vi "XOR Plain Text with Random String.vi"() -> ()   [LabVIEW 2016]
panel:
  out "Plaintext Distribution":dynamicdata(graph)=[{"t0"=timestamp(0.5 s since 1904-01-01), "dt"=1.0, "Y"=[0.0, 0.0, 0.0, 0.0, 0.0, 0.0, 0.0, 0.0, 0.0, 0.0, 0.0, 0.0, 0.0, 0.0, 0.0, 0.0, 0.0, 0.0, 0.0, 0.0, 0.0, 0.0, 0.0, 0.0, 0.0, 0.0, 0.0, 0.0, 0.0, 0.0, 0.0, 0.0, 68.0, 0.0, 0.0, 0.0, 0.0, 0.0, 0.0, 0.0, 0.0, 0.0, 0.0, 0.0, 4.0, 0.0, 4.0, 0.0, 0.0, 0.0, 0.0, 0.0, 0.0, 0.0, 0.0, 0.0, 0.0, 0.0, 0.0, 0.0, 0.0, 0.0, 0.0, 0.0, 0.0, 0.0, 0.0, 0.0, 2.0, 0.0, 0.0, 0.0, 0.0, 0.0, 0.0, 0.0, 1.0, 0.0, 0.0, 0.0, 0.0, 0.0, 0.0, 0.0, 1.0, 0.0, 0.0, 0.0, 0.0, 0.0, 0.0, 0.0, 0.0, 0.0, 0.0, 0.0, 29.0, 0.0, 19.0, 0.0, 55.0, 0.0, 6.0, 0.0, 43.0, 0.0, 0.0, 0.0, 38.0, 0.0, 53.0, 0.0, 16.0, 0.0, 40.0, 0.0, 60.0, 0.0, 3.0, 0.0, 3.0, 0.0, 0.0, 0.0, 0.0, 0.0, 0.0, 0.0, 0.0, 0.0, 0.0, 0.0, 0.0, 0.0, 0.0, 0.0, 0.0, 0.0, 0.0, 0.0, 0.0, 0.0, 0.0, 0.0, 0.0, 0.0, 0.0, 0.0, 0.0, 0.0, 0.0, 0.0, 0.0, 0.0, 0.0, 0.0, 0.0, 0.0, 0.0, 0.0, 0.0, 0.0, 0.0, 0.0, 0.0, 0.0, 0.0, 0.0, 0.0, 0.0, 0.0, 0.0, 0.0, 0.0, 0.0, 0.0, 0.0, 0.0, 0.0, 0.0, 0.0, 0.0, 0.0, 0.0, 0.0, 0.0, 0.0, 0.0, 0.0, 0.0, 0.0, 0.0, 0.0, 0.0, 0.0, 0.0, 0.0, 0.0, 0.0, 0.0, 0.0, 0.0, 0.0, 0.0, 0.0, 0.0, 0.0, 0.0, 0.0, 0.0, 0.0, 0.0, 0.0, 0.0, 0.0, 0.0, 0.0, 0.0, 0.0, 0.0, 0.0, 0.0, 0.0, 0.0, 0.0, 0.0, 0.0, 0.0, 0.0, 0.0, 0.0, 0.0, 0.0, 0.0, 0.0, 0.0, 0.0, 0.0, 0.0, 0.0, 0.0, 0.0, 0.0, 0.0, 0.0, 0.0, 0.0, 0.0, 0.0, 0.0, 0.0, 0.0, 0.0, 0.0, 0.0, 0.0], "attributes"=variant("NI_ChannelName"=variant(string " (Histogram)"), "NI_ExpIsRelativeTime"=variant(bool TRUE), "NI_ExpStartTimeStamp"=variant(timestamp timestamp(3588586549.4751897 s since 1904-01-01)), "NI_ExpTimeStamp"=variant(timestamp timestamp(3588586549.4751897 s since 1904-01-01)), "NI_ExpXDimension"=variant(string "BIN"), "NI_OriginalChannelName"=variant(string ""))}] caption="Histogram"
  out "Cipher Distribution":dynamicdata(graph)=[{"t0"=timestamp(0.5 s since 1904-01-01), "dt"=1.0, "Y"=[5.0, 0.0, 5.0, 0.0, 6.0, 0.0, 6.0, 0.0, 4.0, 0.0, 3.0, 0.0, 4.0, 0.0, 8.0, 0.0, 2.0, 0.0, 3.0, 0.0, 1.0, 0.0, 5.0, 0.0, 5.0, 0.0, 5.0, 0.0, 4.0, 0.0, 1.0, 0.0, 2.0, 0.0, 5.0, 0.0, 4.0, 0.0, 2.0, 0.0, 3.0, 0.0, 3.0, 0.0, 2.0, 0.0, 4.0, 0.0, 6.0, 0.0, 4.0, 0.0, 4.0, 0.0, 5.0, 0.0, 3.0, 0.0, 2.0, 0.0, 2.0, 0.0, 10.0, 0.0, 10.0, 0.0, 9.0, 0.0, 4.0, 0.0, 3.0, 0.0, 3.0, 0.0, 3.0, 0.0, 3.0, 0.0, 2.0, 0.0, 8.0, 0.0, 2.0, 0.0, 3.0, 0.0, 2.0, 0.0, 0.0, 0.0, 4.0, 0.0, 3.0, 0.0, 3.0, 0.0, 3.0, 0.0, 3.0, 0.0, 0.0, 0.0, 5.0, 0.0, 2.0, 0.0, 2.0, 0.0, 3.0, 0.0, 7.0, 0.0, 1.0, 0.0, 2.0, 0.0, 3.0, 0.0, 4.0, 0.0, 5.0, 0.0, 4.0, 0.0, 3.0, 0.0, 2.0, 0.0, 2.0, 0.0, 0.0, 0.0, 6.0, 0.0, 2.0, 0.0, 5.0, 0.0, 0.0, 0.0, 4.0, 0.0, 2.0, 0.0, 4.0, 0.0, 6.0, 0.0, 0.0, 0.0, 5.0, 0.0, 3.0, 0.0, 2.0, 0.0, 1.0, 0.0, 4.0, 0.0, 3.0, 0.0, 4.0, 0.0, 4.0, 0.0, 3.0, 0.0, 1.0, 0.0, 4.0, 0.0, 6.0, 0.0, 3.0, 0.0, 4.0, 0.0, 4.0, 0.0, 5.0, 0.0, 5.0, 0.0, 1.0, 0.0, 1.0, 0.0, 4.0, 0.0, 3.0, 0.0, 2.0, 0.0, 3.0, 0.0, 5.0, 0.0, 4.0, 0.0, 6.0, 0.0, 4.0, 0.0, 4.0, 0.0, 1.0, 0.0, 3.0, 0.0, 0.0, 0.0, 1.0, 0.0, 3.0, 0.0, 4.0, 0.0, 4.0, 0.0, 4.0, 0.0, 3.0, 0.0, 4.0, 0.0, 5.0, 0.0, 3.0, 0.0, 3.0, 0.0, 3.0, 0.0, 4.0, 0.0, 3.0, 0.0, 3.0, 0.0, 2.0, 0.0, 1.0, 0.0, 7.0, 0.0, 3.0, 0.0, 4.0, 0.0, 5.0, 0.0, 1.0, 0.0, 3.0, 0.0], "attributes"=variant("NI_ChannelName"=variant(string " (Histogram)"), "NI_ExpIsRelativeTime"=variant(bool TRUE), "NI_ExpStartTimeStamp"=variant(timestamp timestamp(3588586549.4751897 s since 1904-01-01)), "NI_ExpTimeStamp"=variant(timestamp timestamp(3588586549.4751897 s since 1904-01-01)), "NI_ExpXDimension"=variant(string "BIN"), "NI_OriginalChannelName"=variant(string ""))}] caption="Histogram"
  out "Key Distribution":dynamicdata(graph)=[{"t0"=timestamp(0.5 s since 1904-01-01), "dt"=1.0, "Y"=[5.0, 0.0, 5.0, 0.0, 2.0, 0.0, 2.0, 0.0, 3.0, 0.0, 4.0, 0.0, 3.0, 0.0, 1.0, 0.0, 2.0, 0.0, 4.0, 0.0, 6.0, 0.0, 2.0, 0.0, 1.0, 0.0, 1.0, 0.0, 4.0, 0.0, 5.0, 0.0, 5.0, 0.0, 5.0, 0.0, 4.0, 0.0, 1.0, 0.0, 6.0, 0.0, 4.0, 0.0, 5.0, 0.0, 3.0, 0.0, 6.0, 0.0, 2.0, 0.0, 2.0, 0.0, 0.0, 0.0, 3.0, 0.0, 4.0, 0.0, 2.0, 0.0, 4.0, 0.0, 4.0, 0.0, 5.0, 0.0, 2.0, 0.0, 3.0, 0.0, 3.0, 0.0, 0.0, 0.0, 3.0, 0.0, 5.0, 0.0, 1.0, 0.0, 0.0, 0.0, 1.0, 0.0, 6.0, 0.0, 4.0, 0.0, 9.0, 0.0, 7.0, 0.0, 6.0, 0.0, 6.0, 0.0, 5.0, 0.0, 6.0, 0.0, 1.0, 0.0, 8.0, 0.0, 4.0, 0.0, 5.0, 0.0, 3.0, 0.0, 6.0, 0.0, 7.0, 0.0, 7.0, 0.0, 4.0, 0.0, 4.0, 0.0, 0.0, 0.0, 5.0, 0.0, 3.0, 0.0, 1.0, 0.0, 5.0, 0.0, 4.0, 0.0, 2.0, 0.0, 3.0, 0.0, 5.0, 0.0, 5.0, 0.0, 3.0, 0.0, 5.0, 0.0, 1.0, 0.0, 3.0, 0.0, 2.0, 0.0, 3.0, 0.0, 6.0, 0.0, 2.0, 0.0, 4.0, 0.0, 4.0, 0.0, 3.0, 0.0, 1.0, 0.0, 4.0, 0.0, 3.0, 0.0, 3.0, 0.0, 5.0, 0.0, 2.0, 0.0, 1.0, 0.0, 3.0, 0.0, 4.0, 0.0, 3.0, 0.0, 2.0, 0.0, 1.0, 0.0, 4.0, 0.0, 3.0, 0.0, 6.0, 0.0, 2.0, 0.0, 8.0, 0.0, 1.0, 0.0, 4.0, 0.0, 2.0, 0.0, 2.0, 0.0, 2.0, 0.0, 6.0, 0.0, 3.0, 0.0, 2.0, 0.0, 3.0, 0.0, 5.0, 0.0, 2.0, 0.0, 3.0, 0.0, 5.0, 0.0, 3.0, 0.0, 5.0, 0.0, 2.0, 0.0, 1.0, 0.0, 3.0, 0.0, 3.0, 0.0, 3.0, 0.0, 0.0, 0.0, 4.0, 0.0, 4.0, 0.0, 4.0, 0.0, 6.0, 0.0, 3.0, 0.0, 4.0, 0.0, 4.0, 0.0, 1.0, 0.0], "attributes"=variant("NI_ChannelName"=variant(string " (Histogram)"), "NI_ExpIsRelativeTime"=variant(bool TRUE), "NI_ExpStartTimeStamp"=variant(timestamp timestamp(3588586549.4751897 s since 1904-01-01)), "NI_ExpTimeStamp"=variant(timestamp timestamp(3588586549.4751897 s since 1904-01-01)), "NI_ExpXDimension"=variant(string "BIN"), "NI_OriginalChannelName"=variant(string ""))}] caption="Histogram"
  out "Dechipered":bool=TRUE
  out "Deciphered Text":string="Lorem ipsum dolor sit amet, consectetur adipiscing elit, sed do eiusmod tempor incididunt ut labore et dolore magna aliqua. Ut enim ad minim veniam, quis nostrud exercitation ullamco laboris nisi ut aliquip ex ea commodo consequat. Duis aute irure dolor in reprehenderit in voluptate velit esse cillum dolore eu fugiat nulla pariatur. Excepteur sint occaecat cupidatat non proident, sunt in culpa qui officia deserunt mollit anim id est laborum."
  out "Cipher Text":string
  in  "Plain Text":string="Lorem ipsum dolor sit amet, consectetur adipiscing elit, sed do eiusmod tempor incididunt ut labore et dolore magna aliqua. Ut enim ad minim veniam, quis nostrud exercitation ullamco laboris nisi ut aliquip ex ea commodo consequat. Duis aute irure dolor in reprehenderit in voluptate velit esse cillum dolore eu fugiat nulla pariatur. Excepteur sint occaecat cupidatat non proident, sunt in culpa qui officia deserunt mollit anim id est laborum."
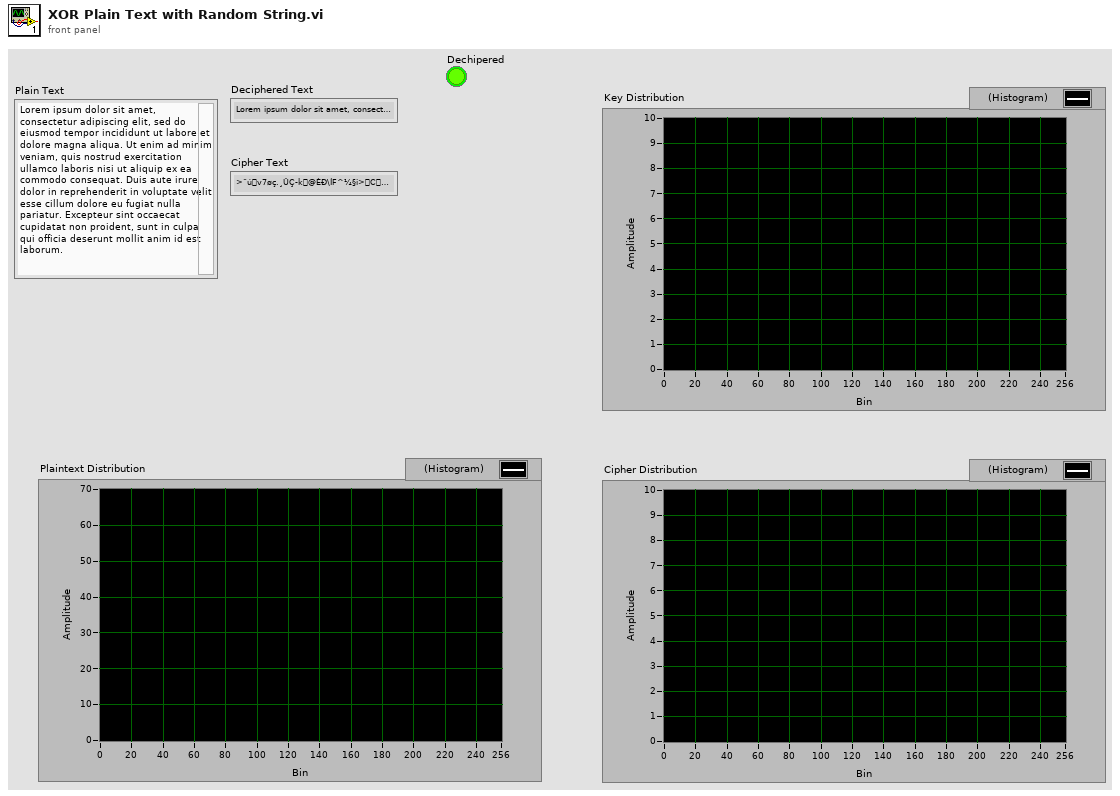
[diagram p1: front panel]
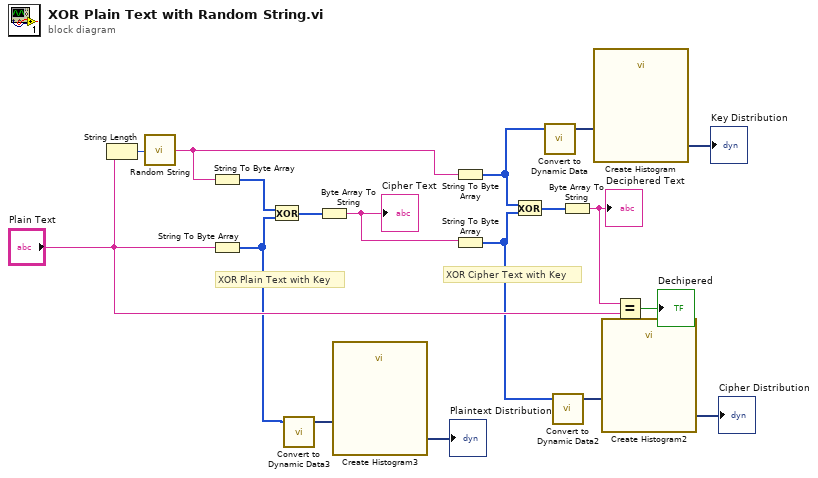
[diagram p0: block diagram]
diagram:
  # "XOR Cipher Text with Key"
  # "XOR Plain Text with Key"
  n1 = String Length(string="Plain Text") -> (length=w13:i32)
  n2 = call "Random String.vi"("length"=w13) -> ("random data"=w14:string)  [unwired: 4 in]
  n3 = String To Byte Array(string=w14) -> (unsigned byte array=w18:u8[])
  n4 = String To Byte Array(string="Plain Text") -> (unsigned byte array=w1:u8[])
  n5 = Exclusive Or(1:w1, 2:w18) -> (0:w17:u8[])
  n6 = call "Convert to Dynamic Data3"("Array"=w1) -> ("Dynamic Data Type"=w3:dynamicdata)  [unwired: 3 in]
  n7 = Byte Array To String(unsigned byte array=w17) -> (string=w15:string)
  "Cipher Text" <- w15
  n8 = call "Create Histogram3"("Signal"=w3) -> ("Histogram"=→"Plaintext Distribution":dynamicdata)  [unwired: 9 in, 1 out]
  n9 = String To Byte Array(string=w14) -> (unsigned byte array=w9:u8[])
  n10 = String To Byte Array(string=w15) -> (unsigned byte array=w4:u8[])
  n11 = Exclusive Or(1:w4, 2:w9) -> (0:w16:u8[])
  n12 = call "Convert to Dynamic Data"("Array"=w9) -> ("Dynamic Data Type"=w8:dynamicdata)  [unwired: 3 in]
  n13 = call "Convert to Dynamic Data2"("Array"=w4) -> ("Dynamic Data Type"=w5:dynamicdata)  [unwired: 3 in]
  n14 = Byte Array To String(unsigned byte array=w16) -> (string=w12:string)
  "Deciphered Text" <- w12
  n15 = call "Create Histogram"("Signal"=w8) -> ("Histogram"=→"Key Distribution":dynamicdata)  [unwired: 9 in, 1 out]
  n16 = call "Create Histogram2"("Signal"=w5) -> ("Histogram"=→"Cipher Distribution":dynamicdata)  [unwired: 9 in, 1 out]
  n17 = Equal?(x=w12, y="Plain Text") -> (x = y?=→"Dechipered":bool)
